vi "LPT-GUI-MIC-ver 5c GLOBAL 1.0.vi"() -> ()   [LabVIEW 2019]
panel:
  in  "SHUTDOWN\nPROGRAM":bool
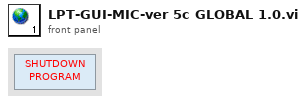
[diagram p1: front panel]
diagram:
